vi "obj_DataLog Aggregation Buffer.vi"(0 "method":T2, 7 "point":T1 {"value" format="%.3e"; "time" format="%<%H:%M:%S%2u\n%Y/%m/%d>T"}, 9 "tag index":i32=-1, 11 "error in (no error)":errorcluster, 12 "aggregation capacity {initialize}":i32, 13 "aggregation fraction {initialize}":dbl format="%.2f") -> (4 "flush needed?":bool, 15 "error out":errorcluster)   [LabVIEW 2012]
doc: "This buffer object aggregates the reduced point data of the various tags that need logging. By regularly updating an on-disk copy of this buffer (the recovery file), the data to be logged is comitted to permanent storage very quickly, safeguarding it from oblivion in case of a power outage or crash, while only having to update a single file. This together with the large buffer size makes that a very leasurely approach can be taken to flushing the per-tag data out to the individual on-disk tag logs (which requires latency-limited multi-file access). During recovery, the recovery file is used to rebuild the aggregation buffer state after which the as yet unflushed data is flush to the various tag logs.\n\nThe flushing methods are inert when this object is not initialized. This safeguard is required because these methods might be called from outside logging runlevel tasks, e.g. the automatic flush when a tag's disk log is queried.\n\nA special {write special} method is provided for logging algorithms that can involve a long latency before a point is actually logged. Such writes are not logged but ensure the availability of recent data during a recovery so that the tag logs can be properly terminated with recent points.\n\nA number of in-memory data structures are maintained to ensure that flushing a particular tag as well as finding the oldest unflushed tag are O(1) operations in the number of tags and buffer size."
uses:
  typedefs/t_DataLog Aggregation Buffer Methods.ctl
  typedefs/clusters/t_DataLog Point.ctl
  typedefs/clusters/t_DataLog Aggregation Entry.ctl
  typedefs/t_DataLog Flush List Methods.ctl
  typedefs/t_DataLog Tag Hash Methods.ctl
  subvis/private/glb_DataLog Runtime Parameterisation.vi
  subvis/private/glb_DataLog MCVD.vi
panel:
  out "dup tag index":i32
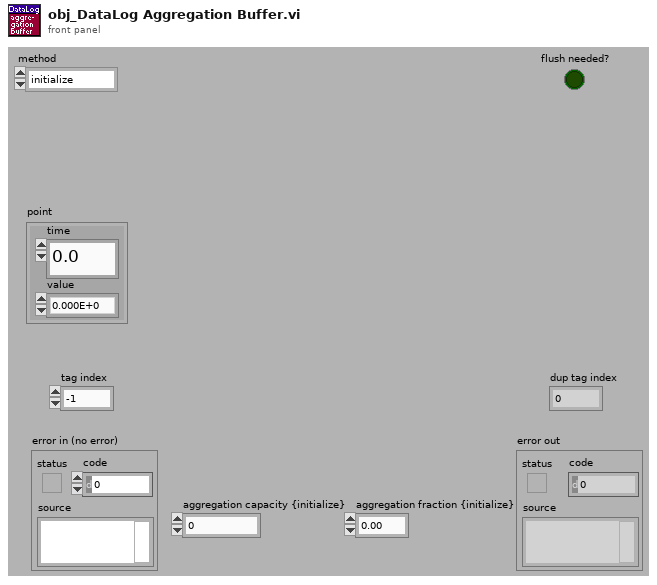
[diagram p1: front panel]
types:
  T1 = typedef "t_DataLog Point.ctl" = cluster{"time":dbl, "value":dbl}
  T2 = typedef "t_DataLog Aggregation Buffer Methods.ctl" = enum16{"initialize", "write", "write special", "flush", "flush next", "flush next if", "setup recovery", "update recovery", "verify recovery", "dummy flush ", "cleanup"}
  T3 = typedef "t_DataLog Aggregation Entry.ctl" = cluster{"tag index":i32, "point":T1}
  T4 = typedef "t_DataLog Flush List Methods.ctl" = enum16{"initialize", "add", "remove", "remove next", "info", "info of next", "cleanup"}
  T5 = typedef "t_DataLog Tag Hash Methods.ctl" = enum16{"initialize", "add tag", "index tag", "lookup", "#tags", "cleanup", "write recovery", "read recovery", "delete recovery"}
  T6 = enum16{"deny read/write", "deny write-only", "deny none"}
  T7 = enum16{"read/write", "read-only", "write-only", "write-only (truncate)"}
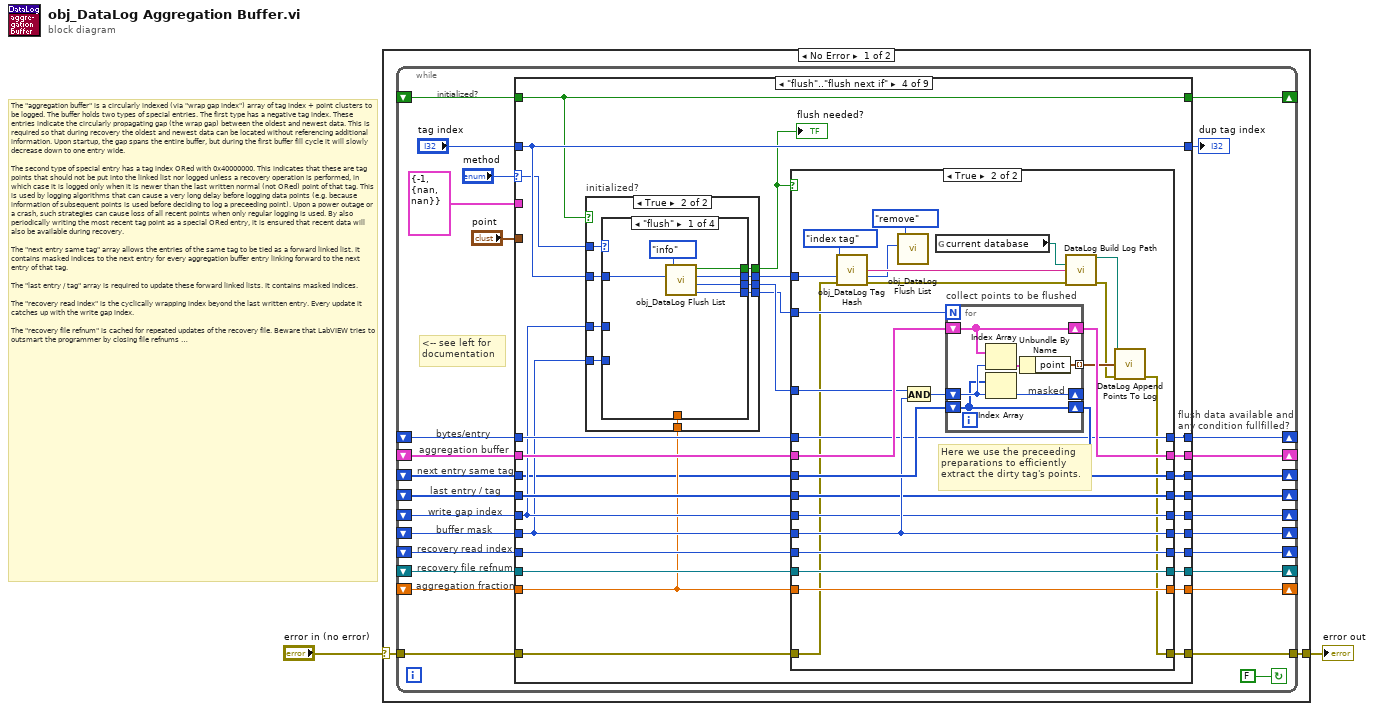
[diagram p0: block diagram]
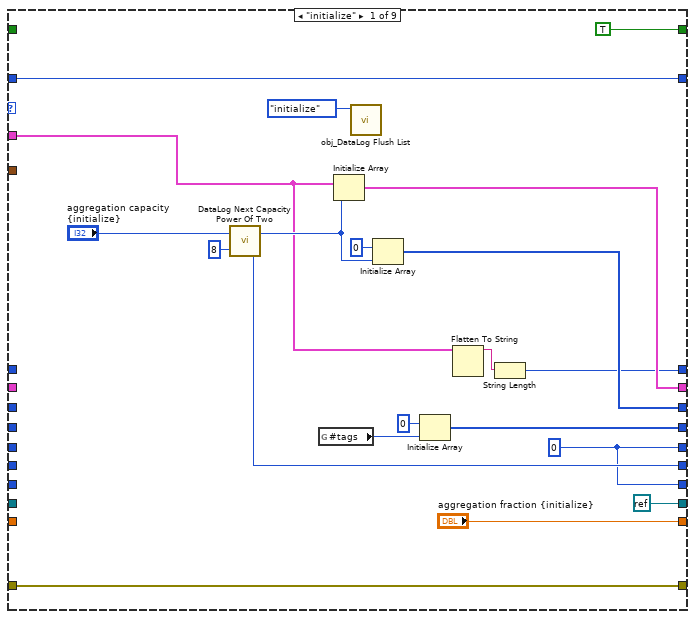
[diagram p2: hidden frame]
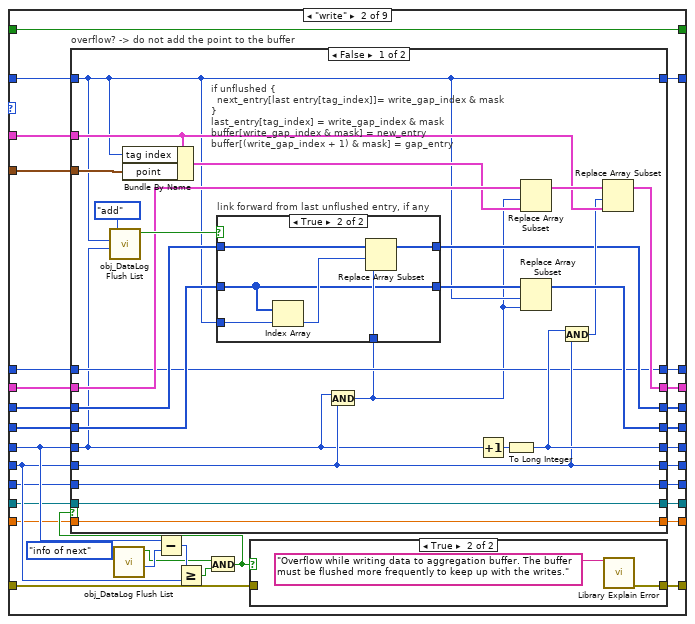
[diagram p3: hidden frame]
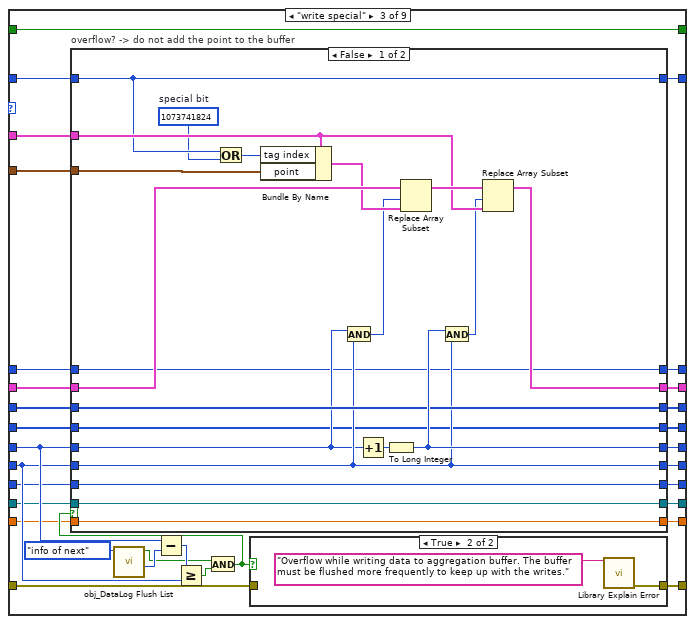
[diagram p7: hidden frame]
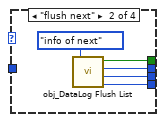
[diagram p11: hidden frame]
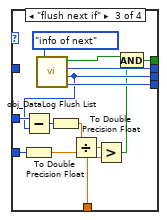
[diagram p12: hidden frame]
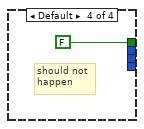
[diagram p13: hidden frame]
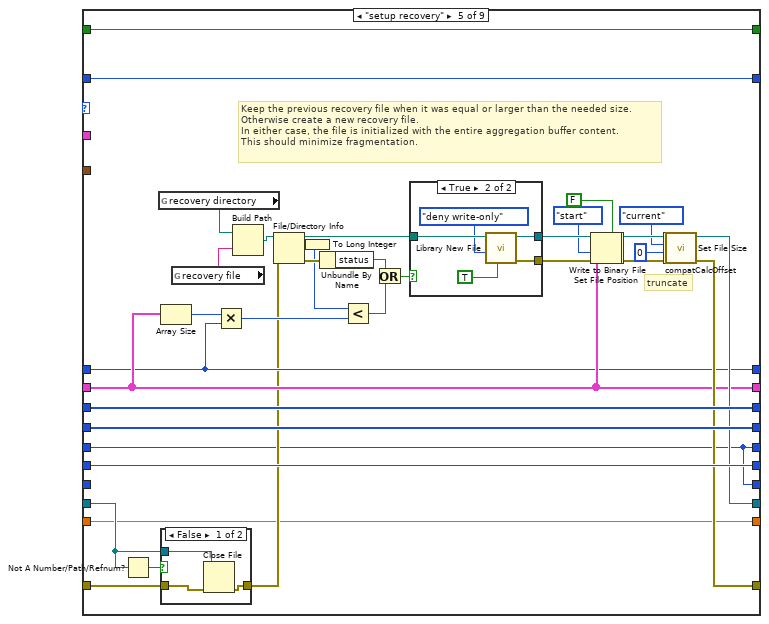
[diagram p15: hidden frame]
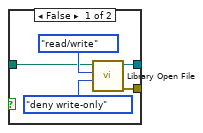
[diagram p17: hidden frame]
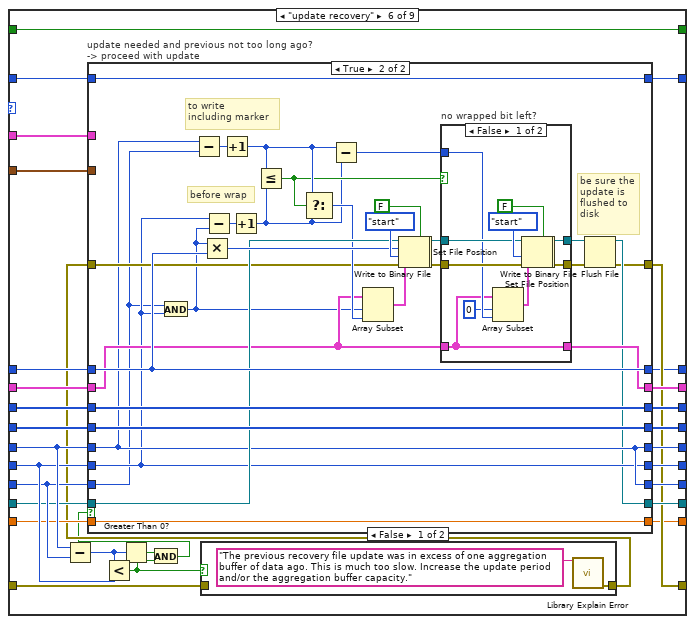
[diagram p18: hidden frame]
diagram:
  # "The \"aggregation buffer\" is a circularly indexed (via \"wrap gap index\") array of tag index + point clusters to be logged. The buffer holds two types of special entries. The first type has a negative tag index. These entries indicate the circularly propagating gap (the wrap gap) between the oldest and newest data. This is required so that during recovery the oldest and newest data can be located without referencing additional information. Upon startup, the gap spans the entire buffer, but during the first buffer fill cycle it will slowly decrease down to one entry wide.\n\nThe second type of special entry has a tag index ORed with 0x40000000. This indicates that these are tag points that should not be put into the linked list nor logged unless a recovery operation is performed, in which case it is logged only when it is newer than the last written normal (not ORed) point of that tag. This is used by logging algorithms that can cause a very long delay before logging data points (e.g. because information of subsequent points is used before deciding to log a preceeding point). Upon a power outage or a crash, such strategies can cause loss of all recent points when only regular logging is used. By also periodically writing the most recent tag point as a special ORed entry, it is ensured that recent data will also be available during recovery.\n\nThe \"next entry same tag\" array allows the entries of the same tag to be tied as a forward linked list. It contains masked indices to the next entry for every aggregation buffer entry linking forward to the next entry of that tag.\n\nThe \"last entry / tag\" array is required to update these forward linked lists. It contains masked indices.\n\nThe \"recovery read index\" is the cyclically wrapping index beyond the last written entry. Every update it catches up with the write gap index.\n\nThe \"recovery file refnum\" is cached for repeated updates of the recovery file. Beware that LabVIEW tries to outsmart the programmer by closing file refnums held by top level VIs that stop running. Consequently, manual testing of this VI's recovery I/O is not possible."
  n1 = case shown="No Error" "error in (no error)" {
    selector: "error in (no error)" -> [w4 w531]
    tunnel: [w3 w531] -> w1
    frame No Error {
      n2 = while {
        shift-right: [w26] -> _
        shift-left: _ -> [w25]
        shift-right: [w30] -> _
        shift-left: _ -> [w29]
        shift-right: [w27] -> _
        shift-left: _ -> [w28]
        tunnel: w4 -> [w24]
        tunnel: [w11] -> w3
        shift-right: [w22] -> _
        shift-left: _ -> [w23]
        shift-right: [w19] -> _
        shift-left: _ -> [w20]
        shift-right: [w16] -> _
        shift-left: _ -> [w17]
        shift-right: [w14] -> _
        shift-left: _ -> [w15]
        shift-right: [w12] -> _
        shift-left: _ -> [w13]
        shift-right: [w7] -> _
        shift-left: _ -> [w8]
        shift-right: [w6] -> _
        shift-left: _ -> [w5]
        stop <- FALSE continue-if-true
        # "initialized?"
        # "<-- see left for\ndocumentation"
        # "aggregation fraction"
        # "bytes/entry"
        # "recovery file refnum"
        # "recovery read index"
        # "write gap index"
        # "buffer mask"
        # "last entry / tag"
        # "next entry same tag"
        # "aggregation buffer"
        n3 = case shown="\"flush\"..\"flush next if\"" "method" {
          selector: "method" -> [_ _ _ w201 _ _ _ _ _]
          tunnel: w29 -> [_ w82 w158 w218 w320 w380 w455 w499 w511]
          tunnel: [w51 w81 w157 w212 w320 w379 w455 w499 w510] -> w30
          tunnel: w28 -> [_ w72 w148 w195 w336 w374 w477 w503 w514]
          tunnel: [w47 w71 w147 w213 w336 w373 w477 w503 w513] -> w27
          tunnel: [w45 w83 w159 w214 w337 w381 w478 w504 w517] -> w26
          tunnel: w25 -> [_ w79 w155 w217 w337 w377 w478 w504 w518]
          tunnel: [w37 w68 w144 w220 w309 w370 w453 w495 w519] -> w10
          tunnel: w24 -> [w52 w77 w153 w209 w312 w375 w463 w496 w522]
          tunnel: [w52 w76 w152 w204 w321 w363 w473 w496 w525] -> w11
          tunnel: w23 -> [_ w67 w143 w199 w311 w369 w476 w502 _]
          tunnel: [w42 w78 w154 w215 w311 w376 w476 w502 w508] -> w22
          tunnel: "point" -> [_ w69 w145 _ _ w371 _ _ _]
          tunnel: w20 -> [_ w66 w142 w198 w335 w368 w474 w500 _]
          tunnel: [w50 w70 w146 w216 w335 w372 w474 w500 w508] -> w19
          tunnel: T3 {"tag index"=-1, "point"={"time"=nan, "value"=nan}} ("aggregation entry") -> [w38 w80 w156 _ _ w378 w458 _ _]
          tunnel: w17 -> [_ w65 w141 w207 _ w366 w475 w501 _]
          tunnel: [w42 w64 w140 w208 w311 w367 w475 w501 w508] -> w16
          tunnel: w15 -> [_ w63 w139 w206 w314 w365 w465 w497 w521]
          tunnel: [refnum<k0> refnum w62 w138 w205 w322 w364 w471 w497 refnum<k0> refnum] -> w14
          tunnel: w13 -> [_ w61 w137 w219 w316 w362 w460 w498 w520]
          tunnel: [w39 w60 w136 w211 w316 w361 w460 w498 w520] -> w12
          tunnel: "tag index" -> [w37 w56 w132 w220 w309 w360 w453 w495 w519]
          tunnel: w8 -> [_ w55 w131 w196 w307 w359 w452 w494 w509]
          tunnel: ["aggregation fraction {initialize}" w54 w130 w197 w307 w358 w452 w494 w509] -> w7
          tunnel: [TRUE w53 w129 w194 w305 w357 w451 w493 FALSE] -> w6
          tunnel: w5 -> [_ w53 w129 w194 w305 w357 w451 w493 _]
          frame "initialize" {
            w42 = 0 ("mask (2^N-1)")
            n4 = call "DataLog Next Capacity Power Of Two.vi"("lower limit"=8, "min capacity"="aggregation capacity {initialize}") -> ("mask (2^N-1)"=w50:i32, "actual capacity (2^N)"=w49:i32)
            n5 = global read "glb_DataLog Runtime Parameterisation.vi" "#tags"() -> (w34:i32)
            n6 = Initialize Array(w38, w49) -> (w51:T3[])
            n7 = call "obj_DataLog Flush List.vi"("method"=t_DataLog_Flush_List_Methods."initialize") -> ()  [unwired: 3 in, 4 out]
            n8 = Initialize Array(0 ("mask (2^N-1)"), w49) -> (w47:i32[])
            n9 = Initialize Array(0 ("mask (2^N-1)"), w34) -> (w45:i32[])
            n10 = Flatten To String(anything=w38) -> (data string=w40:string)  [unwired: 3 in, 2 out]
            n11 = String Length(string=w40) -> (length=w39:i32)
          }
          frame "write" {
            n12 = call "obj_DataLog Flush List.vi"("method"=t_DataLog_Flush_List_Methods."info of next") -> ("entry index out"=w74:i32, "unflushed?"=w58:bool)  [unwired: 3 in, 2 out]
            n13 = Subtract(x=w67, y=w74) -> (x-y=w73:i32)
            n14 = Greater Or Equal?(x=w73, y=w66) -> (x >= y?=w59:bool)
            n15 = And(x=w58, y=w59) -> (x .and. y?=w57:bool)
            n16 = case "overflow? -> do not add the point to the buffer" shown="False" w57 {
              tunnel: [w106 w123] -> w83
              tunnel: w82 -> [w104 w125]
              tunnel: [w101 w125] -> w81
              tunnel: w80 -> [w100 _]
              tunnel: w79 -> [w99 w123]
              tunnel: [w96 w122] -> w78
              tunnel: w56 -> [w90 w120]
              tunnel: w72 -> [w95 w124]
              tunnel: [w94 w124] -> w71
              tunnel: [w93 w121] -> w70
              tunnel: w66 -> [w93 w121]
              tunnel: w69 -> [w92 _]
              tunnel: w67 -> [w86 w122]
              tunnel: [w90 w120] -> w68
              tunnel: w65 -> [w89 w119]
              tunnel: [w89 w119] -> w64
              tunnel: w63 -> [w88 w118]
              tunnel: [w88 w118] -> w62
              tunnel: w61 -> [w87 w117]
              tunnel: [w87 w117] -> w60
              tunnel: w55 -> [w84 w116]
              tunnel: [w84 w116] -> w54
              frame False {
                # "if unflushed {\n  next_entry[last entry[tag_index]]= write_gap_index & mask\n}\nlast_entry[tag_index] = write_gap_index & mask\nbuffer[write_gap_index & mask] = new_entry\nbuffer[(write_gap_index + 1) & mask] = gap_entry"
                n17 = call "obj_DataLog Flush List.vi"("entry index in"=w86, "tag index in"=w90, "method"=t_DataLog_Flush_List_Methods."add") -> ("unflushed?"=w105:bool)  [unwired: 1 in, 3 out]
                n18 = Bundle By Name(cluster=w100, "tag index"=w90, "point"=w92) -> (w103:T3)
                n19 = And(x=w86, y=w93) -> (x .and. y?=w85:i32)
                n20 = case "link forward from last unflushed entry, if any" shown="True" w105 {
                  tunnel: w99 -> [w108 w110]
                  tunnel: w90 -> [_ w115]
                  tunnel: w85 -> [_ w113]
                  tunnel: [w109 w112] -> w94
                  tunnel: w95 -> [w109 w111]
                  tunnel: [w108 w110] -> w91
                  frame False {
                  }
                  frame True {
                    n21 = Index Array(array=w110, index=w115) -> (element=w114:i32)
                    n22 = Replace Array Subset(array=w111, new element=w113, index=w114) -> (w112:i32[])
                  }
                }
                n23 = Increment(x=w86) -> (x+1=w97:i32)
                n24 = To Long Integer(number=w97) -> (32bit integer=w96:i32)
                n25 = Replace Array Subset(array=w104, new element=w103, index=w85) -> (w102:T3[])
                n26 = Replace Array Subset(array=w91, new element=w85, index=w90) -> (w106:i32[])
                n27 = And(x=w96, y=w93) -> (x .and. y?=w98:i32)
                n28 = Replace Array Subset(array=w102, new element=w100, index=w98) -> (w101:T3[])
              }
              frame True {
              }
            }
            n29 = case shown="True" w57 {
              tunnel: w77 -> [w126 _]
              tunnel: [w126 w128] -> w76
              frame False {
              }
              frame True {
                n30 = call "Library Explain Error.vi"("explanation prefix (none)"="Overflow while writing data to aggregation buffer. The buffer must be flushed more frequently to keep up with the writes." ("explanation")) -> ("explained error"=w128:errorcluster)  [unwired: 14 in]
              }
            }
          }
          frame "write special" {
            n31 = call "obj_DataLog Flush List.vi"("method"=t_DataLog_Flush_List_Methods."info of next") -> ("entry index out"=w150:i32, "unflushed?"=w134:bool)  [unwired: 3 in, 2 out]
            n32 = Subtract(x=w143, y=w150) -> (x-y=w149:i32)
            n33 = Greater Or Equal?(x=w149, y=w142) -> (x >= y?=w135:bool)
            n34 = And(x=w134, y=w135) -> (x .and. y?=w133:bool)
            n35 = case "overflow? -> do not add the point to the buffer" shown="False" w133 {
              tunnel: [w162 w188] -> w159
              tunnel: w158 -> [w180 w190]
              tunnel: [w177 w190] -> w157
              tunnel: w156 -> [w176 _]
              tunnel: w155 -> [w162 w188]
              tunnel: [w173 w187] -> w154
              tunnel: w132 -> [w167 w185]
              tunnel: w148 -> [w172 w189]
              tunnel: [w172 w189] -> w147
              tunnel: [w171 w186] -> w146
              tunnel: w142 -> [w171 w186]
              tunnel: w145 -> [w170 _]
              tunnel: w143 -> [w168 w187]
              tunnel: [w167 w185] -> w144
              tunnel: w141 -> [w166 w184]
              tunnel: [w166 w184] -> w140
              tunnel: w139 -> [w165 w183]
              tunnel: [w165 w183] -> w138
              tunnel: w137 -> [w164 w182]
              tunnel: [w164 w182] -> w136
              tunnel: w131 -> [w160 w181]
              tunnel: [w160 w181] -> w130
              frame False {
                w161 = 1073741824  # special bit
                n36 = Or(x=w167, y=w161) -> (x .or. y?=w163:i32)
                n37 = Bundle By Name(cluster=w176, "tag index"=w163, "point"=w170) -> (w179:T3)
                n38 = And(x=w168, y=w171) -> (x .and. y?=w169:i32)
                n39 = Increment(x=w168) -> (x+1=w174:i32)
                n40 = To Long Integer(number=w174) -> (32bit integer=w173:i32)
                n41 = Replace Array Subset(array=w180, new element=w179, index=w169) -> (w178:T3[])
                n42 = And(x=w173, y=w171) -> (x .and. y?=w175:i32)
                n43 = Replace Array Subset(array=w178, new element=w176, index=w175) -> (w177:T3[])
              }
              frame True {
              }
            }
            n44 = case shown="True" w133 {
              tunnel: w153 -> [w191 _]
              tunnel: [w191 w193] -> w152
              frame False {
              }
              frame True {
                n45 = call "Library Explain Error.vi"("explanation prefix (none)"="Overflow while writing data to aggregation buffer. The buffer must be flushed more frequently to keep up with the writes." ("explanation")) -> ("explained error"=w193:errorcluster)  [unwired: 14 in]
              }
            }
          }
          frame "flush".."flush next if" {
            n46 = case "initialized?" shown="True" w194 {
              tunnel: w220 -> [_ w229]
              tunnel: [_ w228] -> w210
              tunnel: [_ w227] -> w203
              tunnel: [_ w226] -> w202
              tunnel: w201 -> [_ w225]
              tunnel: [_ w224] -> w200
              tunnel: w199 -> [_ w223]
              tunnel: w198 -> [_ w222]
              tunnel: w196 -> [_ w221]
              frame False {
              }
              frame True {
                n47 = case shown="\"flush\"" w225 {
                  tunnel: w229 -> [w234 _ _ _]
                  tunnel: [w233 w239 w253 _] -> w228
                  tunnel: [w232 w238 w251 FALSE ("unflushed?")] -> w224
                  tunnel: [w231 w237 w244 _] -> w227
                  tunnel: [w230 w236 w252 _] -> w226
                  tunnel: w223 -> [_ _ w249 _]
                  tunnel: w222 -> [_ _ w246 _]
                  tunnel: w221 -> [_ _ w241 _]
                  frame "flush" {
                    n48 = call "obj_DataLog Flush List.vi"("tag index in"=w234, "method"=t_DataLog_Flush_List_Methods."info") -> ("entries to flush"=w230:i32, "entry index out"=w231:i32, "tag index out"=w233:i32, "unflushed?"=w232:bool)  [unwired: 2 in]
                  }
                  frame "flush next" {
                    n49 = call "obj_DataLog Flush List.vi"("method"=t_DataLog_Flush_List_Methods."info of next") -> ("entries to flush"=w236:i32, "entry index out"=w237:i32, "tag index out"=w239:i32, "unflushed?"=w238:bool)  [unwired: 3 in]
                  }
                  frame "flush next if" {
                    n50 = To Double Precision Float(number=w246) -> (double precision float=w245:dbl)
                    n51 = call "obj_DataLog Flush List.vi"("method"=t_DataLog_Flush_List_Methods."info of next") -> ("entries to flush"=w252:i32, "entry index out"=w244:i32, "tag index out"=w253:i32, "unflushed?"=w250:bool)  [unwired: 3 in]
                    n52 = Subtract(x=w249, y=w244) -> (x-y=w248:i32)
                    n53 = To Double Precision Float(number=w248) -> (double precision float=w247:dbl)
                    n54 = Divide(x=w247, y=w245) -> (x/y=w243:dbl)
                    n55 = Greater?(x=w243, y=w241) -> (0:w242:bool)
                    n56 = And(x=w250, y=w242) -> (x .and. y?=w251:bool)
                  }
                  frame Default {
                    # "should not\nhappen"
                  }
                }
              }
            }
            "flush needed?" <- w200
            n57 = case "flush data available and any condition fullfilled?" shown="True" w200 {
              tunnel: w219 -> [w265 w284]
              tunnel: w195 -> [w263 w291]
              tunnel: w218 -> [w264 w290]
              tunnel: w217 -> [w262 w287]
              tunnel: w199 -> [w261 w288]
              tunnel: w198 -> [w260 w289]
              tunnel: [w260 w289] -> w216
              tunnel: [w261 w288] -> w215
              tunnel: [w262 w287] -> w214
              tunnel: [w263 w286] -> w213
              tunnel: [w264 w285] -> w212
              tunnel: [w265 w284] -> w211
              tunnel: w210 -> [_ w273]
              tunnel: w209 -> [w257 w274]
              tunnel: [w259 w283] -> w208
              tunnel: w207 -> [w259 w283]
              tunnel: w206 -> [w258 w282]
              tunnel: [w258 w282] -> w205
              tunnel: [w257 w276] -> w204
              tunnel: w203 -> [_ w281]
              tunnel: w202 -> [_ w280]
              tunnel: w196 -> [w256 w279]
              tunnel: [w256 w279] -> w197
              frame False {
              }
              frame True {
                # "Here we use the preceeding\npreparations to efficiently\nextract the dirty tag's points."
                n58 = call "obj_DataLog Tag Hash.vi"("method"=t_DataLog_Tag_Hash_Methods."index tag", "tag index in"=w273, "error in (no error)"=w274) -> ("tag out"=w270:string, "tag index out"=w266:i32, "error out"=w271:errorcluster)  [unwired: 9 in, 1 out]
                n59 = call "obj_DataLog Flush List.vi"("tag index in"=w266, "method"=t_DataLog_Flush_List_Methods."remove") -> ()  [unwired: 2 in, 4 out]
                n60 = And(x=w281, y=w289) -> (x .and. y?=w277:i32)
                n61 = global read "glb_DataLog Runtime Parameterisation.vi" "current database"() -> (w269:path)
                n62 = for "collect points to be flushed" {
                  N: w280 -> [_]
                  shift-right: [w293] -> _
                  shift-left: w277 -> [w294]
                  shift-right: [w295] -> w285
                  shift-left: w290 -> [w295]
                  shift-right: [w292] -> w286
                  shift-left: w291 -> [w292]
                  tunnel: [w296] -> w278 mode=indexing
                  # "masked"
                  n63 = Index Array(array=w295, index=w294) -> (element=w297:T3)
                  n64 = Index Array(array=w292, index=w294) -> (element=w293:i32)
                  n65 = Unbundle By Name(w297) -> ("point"=w296:T1)
                }
                n66 = call "DataLog Build Log Path.vi"("database path"=w269, "tag"=w270, "error in (no error)"=w271) -> ("tag log directory"=w267:path, "error out"=w268:errorcluster)  [unwired: 11 in]
                n67 = call "DataLog Append Points To Log.vi"("tag log directory"=w267, "points"=w278, "error in (no error)"=w268) -> ("error out"=w276:errorcluster)  [unwired: 11 in, 1 out]
              }
            }
          }
          frame "setup recovery" {
            # "truncate"
            # "Keep the previous recovery file when it was equal or larger than the needed size.\nOtherwise create a new recovery file.\nIn either case, the file is initialized with the entire aggregation buffer content.\nThis should minimize fragmentation."
            n68 = Not A Number/Path/Refnum?(number/path/refnum=w314) -> (NaN/Path/Refnum?=w315:bool)
            n69 = global read "glb_DataLog Runtime Parameterisation.vi" "recovery directory"() -> (w306:path)
            n70 = Array Size(array=w320) -> (size(s)=w317:i32)
            n71 = case shown="False" w315 {
              tunnel: [w340 w341] -> w313
              tunnel: w314 -> [w339 _]
              tunnel: w312 -> [w338 w341]
              frame False {
                n72 = Close File(refnum=w339, error in=w338) -> (error out=w340:errorcluster)  [unwired: 1 out]
              }
              frame True {
              }
            }
            n73 = global read "glb_DataLog MCVD.vi" "recovery file"() -> (w318:string)
            n74 = Multiply(x=w317, y=w316) -> (x*y=w328:i32)
            n75 = Build Path(base path=w306, name or relative path=w318) -> (appended path=w319:path)
            n76 = File/Directory Info(path=w319, error in=w313) -> (path out=w331:path, size=w304:i64, error out=w330:errorcluster)  [unwired: 4 out]
            n77 = To Long Integer(number=w304) -> (32bit integer=w329:i32)
            n78 = Unbundle By Name(w330) -> ("status"=w326:bool)
            n79 = Less?(x=w329, y=w328) -> (x < y?=w327:bool)
            n80 = Or(x=w326, y=w327) -> (x .or. y?=w325:bool)
            n81 = case shown="True" w325 {
              tunnel: [w344 w350] -> w334
              tunnel: [w343 w351] -> w333
              tunnel: w331 -> [w342 w349]
              frame False {
                n82 = call "Library Open File.vi"("deny mode (deny none)"=T6."deny write-only" ("deny mode (2)"), "open mode (read/write)"=T7."read/write" ("open mode (0)"), "file path"=w342) -> ("error out"=w343:errorcluster, "refnum"=w344:refnum<file>)  [unwired: 3 in]
              }
              frame True {
                n83 = call "Library New File.vi"("overwrite (F)"=TRUE, "deny mode (deny none)"=T6."deny write-only" ("deny mode (2)"), "file path"=w349) -> ("error out"=w351:errorcluster, "refnum"=w350:refnum<file>)  [unwired: 7 in]
              }
            }
            n84 = Set File Position(refnum=w334, from (0:start)=enum16{"start", "end", "current"}."start" ("pos mode (0:2)"), error in=w333) -> (refnum out=w300:refnum<file>, error out=w299:errorcluster)  [unwired: 1 in]
            n85 = Write to Binary File(file (use dialog)=w300, data=w320, error in=w299, 5:FALSE ("prepend array or string size? (T)")) -> (refnum out=w323:refnum<file>, error out=w324:errorcluster)  [unwired: 2 in, 1 out]
            n86 = call <vilib>:"compatCalcOffset.vi"("error in"=w324, "pos offset (0)"=0, "pos mode (0:1)"=enum16{"start", "end", "current"}."current", "refnum"=w323) -> ("error out"=w303:errorcluster, "offset"=w302:i32, "dup refnum"=w301:refnum<file>)  [unwired: 5 in]
            n87 = Set File Size(4:w303, 6:w302, 7:w301) -> (0:w321:errorcluster, 3:w322:refnum<file>)
          }
          frame "update recovery" {
            n88 = Subtract(x=w369, y=w366) -> (x-y=w353:i32)
            n89 = Less?(x=w353, y=w368) -> (x < y?=w355:bool)
            n90 = Greater Than 0?(x=w353) -> (x > 0?=w354:bool)
            n91 = And(x=w354, y=w355) -> (x .and. y?=w352:bool)
            n92 = case shown="False" w355 {
              tunnel: w375 -> [_ w442]
              tunnel: [w441 w442] -> w356
              frame False {
                n93 = call "Library Explain Error.vi"("explanation prefix (none)"="The previous recovery file update was in excess of one aggregation buffer of data ago. This is much too slow. Increase the update period and/or the aggregation buffer capacity." ("explanation")) -> ("explained error"=w441:errorcluster)  [unwired: 14 in]
              }
              frame True {
              }
            }
            n94 = case "update needed and previous not too long ago? -> proceed with update" shown="True" w352 {
              tunnel: [w390 w422] -> w381
              tunnel: w380 -> [w392 w407]
              tunnel: [w392 w404] -> w379
              tunnel: w378 -> [_ _]
              tunnel: w377 -> [w390 w422]
              tunnel: [w389 w405] -> w376
              tunnel: w360 -> [w387 w424]
              tunnel: w374 -> [w391 w423]
              tunnel: [w391 w423] -> w373
              tunnel: [w388 w403] -> w372
              tunnel: w368 -> [w388 w403]
              tunnel: w371 -> [_ _]
              tunnel: w369 -> [w389 w405]
              tunnel: [w387 w424] -> w370
              tunnel: w366 -> [w386 w402]
              tunnel: [w386 w405] -> w367
              tunnel: w365 -> [w385 w415]
              tunnel: [w385 w398] -> w364
              tunnel: w356 -> [w383 w408]
              tunnel: [w383 w397] -> w363
              tunnel: [w384 w418] -> w361
              tunnel: w362 -> [w384 w418]
              tunnel: w359 -> [w382 w396]
              tunnel: [w382 w396] -> w358
              frame False {
              }
              frame True {
                # "be sure the\nupdate is\nflushed to\ndisk"
                # "before wrap"
                # "to write\nincluding marker"
                n95 = And(x=w402, y=w403) -> (x .and. y?=w401:i32)
                n96 = Subtract(x=w405, y=w402) -> (x-y=w421:i32)
                n97 = Multiply(x=w401, y=w418) -> (x*y=w417:i32)
                n98 = Subtract(x=w403, y=w401) -> (x-y=w420:i32)
                n99 = Increment(x=w421) -> (x+1=w412:i32)
                n100 = Increment(x=w420) -> (x+1=w409:i32)
                n101 = Less Or Equal?(x=w412, y=w409) -> (x <= y?=w411:bool)
                n102 = Select(t=w412, s=w411, f=w409) -> (s? t:f=w410:i32)
                n103 = Subtract(x=w412, y=w409) -> (x-y=w406:i32)
                n104 = Array Subset(array=w407, index=w401, length=w410) -> (w416:T3[])
                n105 = Set File Position(offset (in bytes) (0)=w417, refnum=w415, from (0:start)=enum16{"start", "end", "current"}."start" ("pos mode (0:2)"), error in=w408) -> (refnum out=w395:refnum<file>, error out=w394:errorcluster)
                n106 = Write to Binary File(file (use dialog)=w395, data=w416, error in=w394, 5:FALSE ("prepend array or string size? (T)")) -> (refnum out=w413:refnum<file>, error out=w414:errorcluster)  [unwired: 2 in, 1 out]
                n107 = case "no wrapped bit left?" shown="False" w411 {
                  tunnel: w414 -> [w435 w438]
                  tunnel: w413 -> [w434 w439]
                  tunnel: [w433 w439] -> w399
                  tunnel: w407 -> [w428 w437]
                  tunnel: w406 -> [w432 _]
                  tunnel: [w429 w438] -> w400
                  tunnel: [w428 w437] -> w404
                  frame False {
                    n108 = Array Subset(array=w428, index=0, length=w432) -> (w430:T3[])
                    n109 = Set File Position(refnum=w434, from (0:start)=enum16{"start", "end", "current"}."start" ("pos mode (0:2)"), error in=w435) -> (refnum out=w427:refnum<file>, error out=w426:errorcluster)  [unwired: 1 in]
                    n110 = Write to Binary File(file (use dialog)=w427, data=w430, error in=w426, 5:FALSE ("prepend array or string size? (T)")) -> (refnum out=w433:refnum<file>, error out=w429:errorcluster)  [unwired: 2 in, 1 out]
                  }
                  frame True {
                  }
                }
                n111 = Flush File(refnum=w399, error in=w400) -> (refnum out=w398:refnum<file>, error out=w397:errorcluster)
              }
            }
          }
          frame "verify recovery" {
            # "This is useful for testing purposes:\nIt can help verify whether the recovery\nfile indeed equals the buffer after\nan update."
            n112 = Set File Position(refnum=w465, from (0:start)=enum16{"start", "end", "current"}."end" ("pos mode (0:2)"), error in=w463) -> (refnum out=w450:refnum<file>, error out=w449:errorcluster)  [unwired: 1 in]
            n113 = Get File Position(4:w449, 7:w450) -> (0:w466:errorcluster, 2:w448:i64, 3:w464:refnum<file>)
            n114 = To Long Integer(number=w448) -> (32bit integer=w461:i32)
            n115 = Quotient & Remainder(x=w461, y=w460) -> (floor(x/y)=w459:i32)  [unwired: 1 out]
            n116 = Set File Position(refnum=w464, from (0:start)=enum16{"start", "end", "current"}."start" ("pos mode (0:2)"), error in=w466) -> (refnum out=w447:refnum<file>, error out=w446:errorcluster)  [unwired: 1 in]
            n117 = Read from Binary File(5:w458, 8:w446, 10:w459, 11:w447) -> (0:w444:errorcluster, 2:w456:T3[], 3:w445:refnum<file>)  [unwired: 2 in, 1 out]
            n118 = Get File Position(4:w444, 7:w445) -> (0:w472:errorcluster, 2:w443:i64, 3:w471:refnum<file>)
            n119 = To Long Integer(number=w443) -> (32bit integer=w469:i32)
            n120 = Array Size(array=w456) -> (size(s)=w468:i32)
            n121 = Array Size(array=w455) -> (size(s)=w467:i32)
            n122 = Equal?(x=w468, y=w467) -> (x = y?=w457:bool)
            n123 = for {
              shift-right: [w481] -> w454
              shift-left: w457 -> [w480]
              tunnel: w456 -> [w484] mode=indexing
              tunnel: w455 -> [w485] mode=indexing
              n124 = Flatten To String(anything=w484) -> (data string=w483:string)  [unwired: 3 in, 2 out]
              n125 = Flatten To String(anything=w485) -> (data string=w482:string)  [unwired: 3 in, 2 out]
              n126 = Equal?(x=w483, y=w482) -> (x = y?=w479:bool)
              n127 = And(x=w479, y=w480) -> (x .and. y?=w481:bool)
            }
            n128 = case shown="No Error" w472 {
              selector: w472 -> [w487 w492]
              tunnel: [w486 w492] -> w473
              tunnel: w454 -> [w488 _]
              tunnel: w469 -> [_ _]
              frame No Error {
                n129 = case "equal?" shown="False" w488 {
                  tunnel: [w490 w491] -> w486
                  tunnel: w487 -> [_ w491]
                  frame False {
                    n130 = call "Library Explain Error.vi"("explanation prefix (none)"="The recovery file differs from the aggregation buffer." ("explanation")) -> ("explained error"=w490:errorcluster)  [unwired: 14 in]
                  }
                  frame True {
                  }
                }
              }
              frame Error {
              }
            }
          }
          frame "dummy flush " {
            # "This is useful for testing purposes:\nIt can prevent an overflow error so that\nrecovery can be tested without actual\nflushing."
            n131 = while "remove all entries from the flush list" {
              stop <- w505 continue-if-true
              n132 = call "obj_DataLog Flush List.vi"("method"=t_DataLog_Flush_List_Methods."remove next") -> ("unflushed?"=w505:bool)  [unwired: 3 in, 3 out]
            }
          }
          frame "cleanup" {
            w508 = 0 ("dimension size")
            n133 = Not A Number/Path/Refnum?(number/path/refnum=w521) -> (NaN/Path/Refnum?=w523:bool)
            n134 = Reshape Array(w511, 0 ("dimension size")) -> (w510:T3[])
            n135 = case shown="False" w523 {
              tunnel: [w529 w530] -> w525
              tunnel: w522 -> [w528 w530]
              tunnel: w521 -> [w527 _]
              frame False {
                n136 = Close File(refnum=w527, error in=w528) -> (error out=w529:errorcluster)  [unwired: 1 out]
              }
              frame True {
              }
            }
            n137 = Reshape Array(w514, 0 ("dimension size")) -> (w513:i32[])
            n138 = call "obj_DataLog Flush List.vi"("method"=t_DataLog_Flush_List_Methods."cleanup") -> ()  [unwired: 3 in, 4 out]
            n139 = Reshape Array(w518, 0 ("dimension size")) -> (w517:i32[])
          }
        }
        "dup tag index" <- w10
      }
    }
    frame Error {
    }
  }
  "error out" <- w1
